vi "oval_main.vi"(7 "Reload":bool, 8 "Error In":errorcluster, 11 "ovalization_data":T1={"AngOval"=[0.0, 60.0, 120.0, 22.5, 45.0, 67.5, 90.0, 112.5, 135.0, 157.5, 180.0], "OvalDiam"=[324.25, 324.6, 324.55, 324.25, 324.55, 324.65, 324.6, 324.65, 324.55, 324.5, 324.4], "Plots"={"Ref"={"X"=[], "Y"=[]}, "Elipse"={"X"=[], "Y"=[]}, "Points"={"X"=[], "Y"=[]}}, "Ampliation"=100.0, "Results"={"MD"=0.0, "mD"=0.0, "Dmed"=0.0, "Oval"=0.0, "ang"=0.0, "X0"=0.0, "Y0"=0.0}, "fit"=[]}) -> (0 "Error Out":errorcluster, 3 "output ovalization_data-out":T1={"AngOval"=[0.0, 60.0, 120.0, 22.5, 45.0, 67.5, 90.0, 112.5, 135.0, 157.5, 180.0], "OvalDiam"=[324.25, 324.6, 324.55, 324.25, 324.55, 324.65, 324.6, 324.65, 324.55, 324.5, 324.4], "Plots"={"Ref"={"X"=[], "Y"=[]}, "Elipse"={"X"=[], "Y"=[]}, "Points"={"X"=[], "Y"=[]}}, "Ampliation"=100.0, "Results"={"MD"=0.0, "mD"=0.0, "Dmed"=0.0, "Oval"=0.0, "ang"=0.0, "X0"=0.0, "Y0"=0.0}, "fit"=[]})   [LabVIEW 2016]
uses:
  ovalization_data.ctl
  <vilib>/Utility/miscctls.llb/LVBoundsTypeDef.ctl
  Report/report_mods.ctl
  ExternalDependencies/AlgenLabVIEW/Code/TypeDefs/basic_config.ctl
  ExternalDependencies/AlgenLabVIEW/Code/TypeDefs/termination_data.ctl
  <vilib>/Analysis/baseanly.llb/Mean (DBL).vi
  <vilib>/Analysis/NI_AALBase.lvlib
panel:
  out "oval_plot":cluster{"X":dbl[], "Y":dbl[]}[](graph) caption="Ovalização"
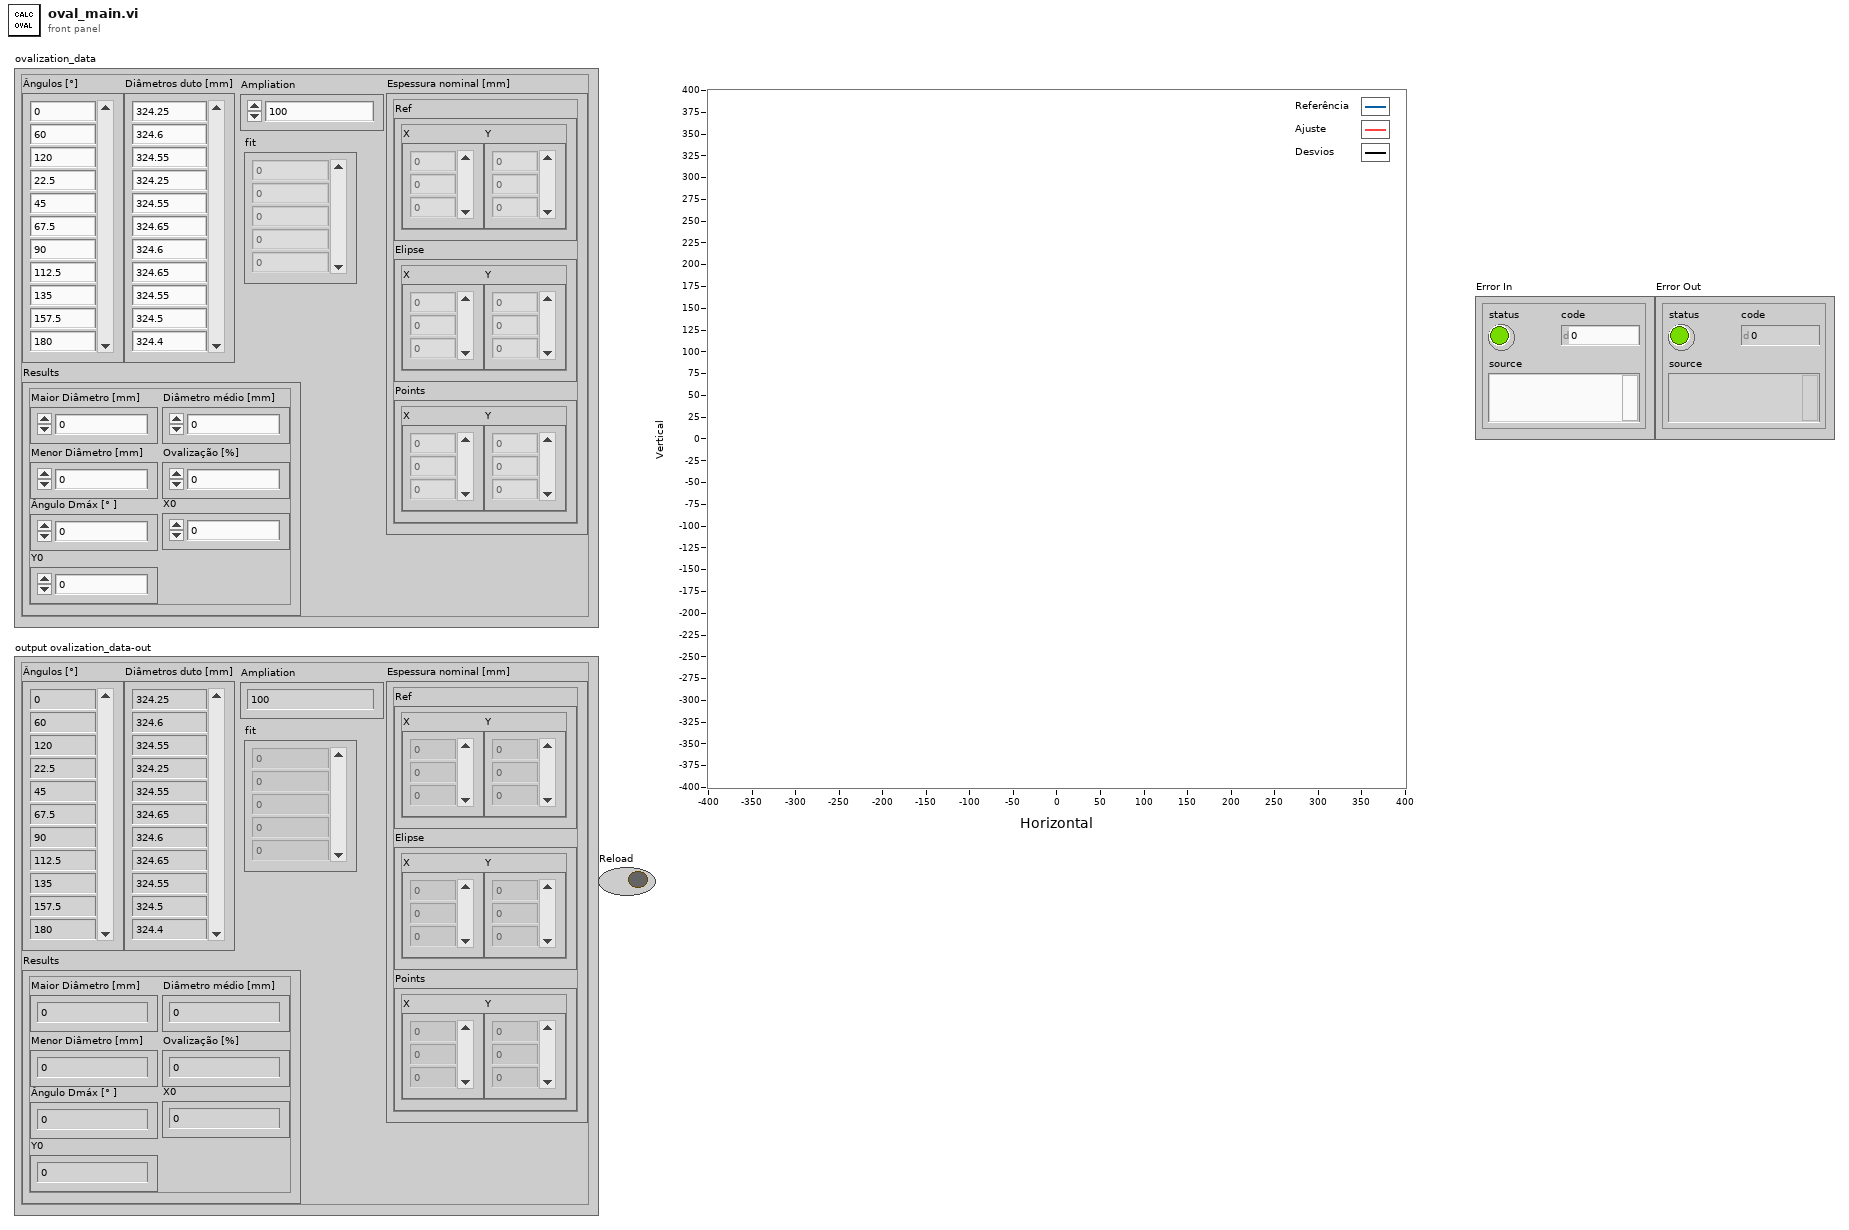
[diagram p1: front panel]
types:
  T1 = typedef "ovalization_data.ctl" = cluster{"AngOval":dbl[], "OvalDiam":dbl[], "Plots":cluster{"Ref":cluster{"X":dbl[], "Y":dbl[]}, "Elipse":cluster{"X":dbl[], "Y":dbl[]}, "Points":cluster{"X":dbl[], "Y":dbl[]}}, "Ampliation":dbl, "Results":cluster{"MD":dbl, "mD":dbl, "Dmed":dbl, "Oval":dbl, "ang":dbl, "X0":dbl, "Y0":dbl}, "fit":dbl[]}
  T2 = typedef "report_mods.ctl" = enum16{"Init", "Table", "Graph", "TablefromGraph", "End"}
  T3 = typedef "LVBoundsTypeDef.ctl" = cluster{"Width":u32, "Height":u32}
  T4 = typedef "termination_data.ctl" = cluster{"MaxGen":cluster{"Generations":i32, "Active":bool}, "CostFunctionTol":cluster{"Tol":dbl, "Active":bool}, "GensEstab":cluster{"Generations":i32, "Active":bool}}
  T5 = typedef "basic_config.ctl" = cluster{"parameters_range":cluster{"Max":dbl, "Min":dbl}[], "Initial elements":i32}
  T6 = typedef "PipePoints.ctl" = cluster{"X":dbl[], "Y":dbl[], "Theta":dbl[]}
  T7 = typedef "GenAlg_data.ctl" = cluster{"BasicCondfig":T5, "elements":T8[], "CostFunction":refnum<vi>, "GenerationData":T9, "SelectionData":T10, "SimulatedAnnealingData":T11, "CostFunctionData":variant, "MultiEval_data":T12, "TerminationData":T4}
  T8 = typedef "element.ctl" = cluster{"Parameters":dbl[], "Cost":dbl}
  T9 = typedef "geration_data.ctl" = cluster{"ElementsCreated":i32}
  T10 = typedef "selection_data.ctl" = cluster{"ElementsSelected":i32}
  T11 = typedef "SimulatedAnnealing_data.ctl" = cluster{"AnnealingFactor":dbl, "Active":bool}
  T12 = typedef "multi_eval_data.ctl" = cluster{"Active":bool, "MultiEvalFunction":refnum<vi>}
  T13 = cluster{"Ref":cluster{"X":dbl[], "Y":dbl[]}, "Elipse":cluster{"X":dbl[], "Y":dbl[]}, "Points":cluster{"X":dbl[], "Y":dbl[]}}
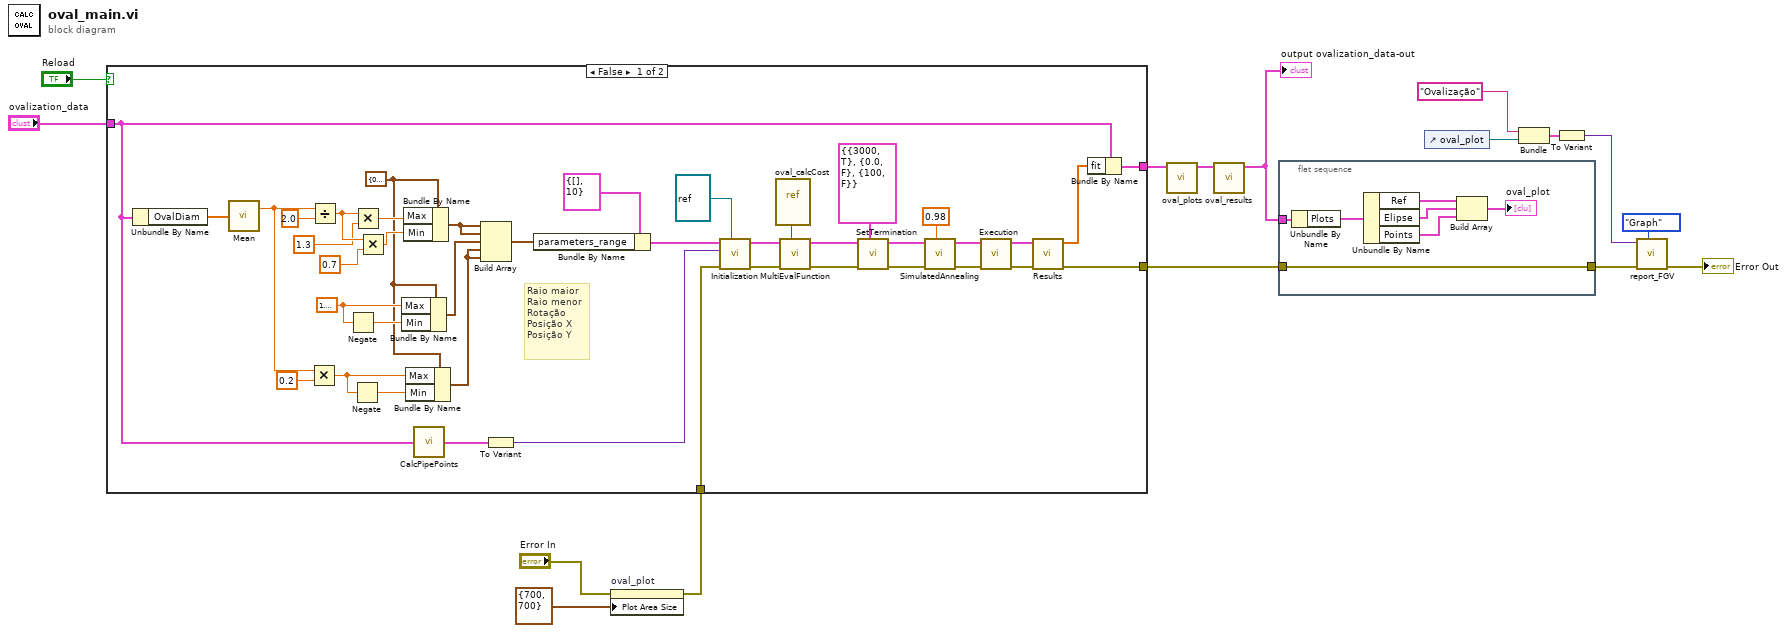
[diagram p0: block diagram]
diagram:
  n1 = property on="oval_plot" class="XYGraph (strict)"(error in="Error In", "Plot Area Size"=T3 {"Width"=700, "Height"=700} ("Plot Area:Size")) -> (error out=w14:errorcluster)  [unwired: 1 in, 1 out]
  n2 = case shown="False" "Reload" {
    tunnel: w14 -> [w21 w58]
    tunnel: [w20 w58] -> w11
    tunnel: "ovalization_data" -> [w19 w59]
    tunnel: [w17 w59] -> w2
    frame False {
      w43 = cluster{"Max":dbl, "Min":dbl} {"Max"=0.0, "Min"=0.0} ("parameters_range")
      w52 = 1.5707963267948966
      # "Raio maior\nRaio menor\nRotação\nPosição X\nPosição Y"
      n3 = Unbundle By Name(w19) -> ("OvalDiam"=w42:dbl[])
      n4 = call-poly <vilib>:"Mean.vi"("X"=w42) -> ("mean"=w41:dbl)  [unwired: 1 out]
      n5 = Multiply(x=w41, y=0.2) -> (x*y=w56:dbl)
      n6 = Divide(x=w41, y=2.0) -> (x/y=w50:dbl)
      n7 = Negate(x=w52) -> (-x=w53:dbl)
      n8 = Negate(x=w56) -> (-x=w55:dbl)
      n9 = Multiply(x=w50, y=1.3) -> (x*y=w47:dbl)
      n10 = Multiply(x=w50, y=0.7) -> (x*y=w48:dbl)
      n11 = Bundle By Name(cluster=w43, "Max"=w52, "Min"=w53) -> (w51:cluster{"Max":dbl, "Min":dbl})
      n12 = Bundle By Name(cluster=w43, "Max"=w47, "Min"=w48) -> (w49:cluster{"Max":dbl, "Min":dbl})
      n13 = Bundle By Name(cluster=w43, "Max"=w56, "Min"=w55) -> (w57:cluster{"Max":dbl, "Min":dbl})
      n14 = call "CalcPipePoints.vi"("ovalization_data"=w19) -> ("PipePoints"=w37:T6)
      n15 = Build Array(w49, w49, w51, w57, w57) -> (w39:cluster{"Max":dbl, "Min":dbl}[])
      n16 = To Variant(anything=w37) -> (Variant=w36:variant)
      n17 = Bundle By Name(cluster=T5 {"parameters_range"=[], "Initial elements"=10} ("basic_config"), "parameters_range"=w39) -> (w38:T5)
      n18 = call "Initialization.vi"("CostFunction"=refnum<vi> refnum, "Error In"=w21, "CostFunctionData"=w36, "basic_config"=w38) -> ("Error Out"=w34:errorcluster, "GenAlg_data"=w29:T7)  [unwired: 6 in]
      n19 = vi-ref "oval_calcCost.vi"() -> (w22:refnum<vi>)
      n20 = call "MultiEvalFunction.vi"("MultiEvalFunction"=w22, "Error In"=w34, "GenAlg_data"=w29) -> ("Error Out"=w33:errorcluster, "GenAlg_data-out"=w28:T7)  [unwired: 7 in]
      n21 = call "SetTermination.vi"("TerminationData"=T4 {"MaxGen"={"Generations"=3000, "Active"=TRUE}, "CostFunctionTol"={"Tol"=0.0, "Active"=FALSE}, "GensEstab"={"Generations"=100, "Active"=FALSE}}, "Error In"=w33, "GenAlg_data"=w28) -> ("Error Out"=w32:errorcluster, "GenAlg_data-out"=w27:T7)  [unwired: 7 in]
      n22 = call "SimulatedAnnealing.vi"("AnnealingFactor"=0.98, "Error In"=w32, "GenAlg_data"=w27) -> ("Error Out"=w31:errorcluster, "GenAlg_data-out"=w26:T7)  [unwired: 7 in]
      n23 = call "Execution.vi"("Error In"=w31, "GenAlg_data"=w26) -> ("Error Out"=w30:errorcluster, "GenAlg_data-out"=w25:T7)  [unwired: 8 in]
      n24 = call "Results.vi"("Error In"=w30, "GenAlg_data"=w25) -> ("Error Out"=w20:errorcluster, "MinPoint"=w18:dbl[])  [unwired: 7 in, 1 out]
      n25 = Bundle By Name(cluster=w19, "fit"=w18) -> (w17:T1)
    }
    frame True {
    }
  }
  n26 = call "oval_plots.vi"("ovalization_data"=w2) -> ("output ovalization_data-out"=w13:T1)  [unwired: 10 in]
  n27 = call "oval_results.vi"("ovalization_data"=w13) -> ("output ovalization_data-out"=w12:T1)  [unwired: 10 in]
  "output ovalization_data-out" <- w12
  n28 = flat-sequence {
    tunnel: w12 -> [w61]
    tunnel: w11 -> [w60]
    tunnel: [w60] -> w10
    frame #0 {
      n29 = Unbundle By Name(w61) -> ("Plots"=w66:T13)
      n30 = Unbundle By Name(w66) -> ("Ref"=w65:cluster{"X":dbl[], "Y":dbl[]}, "Elipse"=w62:cluster{"X":dbl[], "Y":dbl[]}, "Points"=w63:cluster{"X":dbl[], "Y":dbl[]})
      n31 = Build Array(w65, w62, w63) -> (→"oval_plot":cluster{"X":dbl[], "Y":dbl[]}[])
    }
  }
  n32 = control-ref of="oval_plot"() -> (w8:refnum<vi>)
  n33 = Bundle("Ovalização", "oval_plot"=w8) -> (w6:cluster{string, "oval_plot":refnum<vi>})  [unwired: 1 in]
  n34 = To Variant(anything=w6) -> (Variant=w5:variant)
  n35 = call "report_FGV.vi"("report_mods"=report_mods."Graph", "Error In"=w10, "Data in"=w5) -> ("Error Out"=→"Error Out":errorcluster)  [unwired: 8 in]
